vi "Overview Facade.vi"(0 "Data In":T4, 2 "Display State In":T2={"Numeric"=0.0, "Fill Plots"=FALSE, "Cursor Redraw"=TRUE, "XYGraph Refnum"=refnum}, 3 "Container State":T3) -> (6 "Data Out":T4, 7 "Display State Out":T2={"Numeric"=0.0, "Fill Plots"=FALSE, "Cursor Redraw"=TRUE, "XYGraph Refnum"=refnum}, 8 "Action":T1)   [LabVIEW 2020, in "Overview XControl.xctl"]
uses:
  Overview XControl.xctl
  Overview Data.ctl
  <vilib>/_xctls/Container State.ctl
  Overview State.ctl
  <vilib>/_xctls/Action.ctl
  <vilib>/Analysis/2dsp.llb/Decimate (single shot, DBL).vi
  <vilib>/_xctls/XControlSupport.lvlib
  <vilib>/Analysis/NI_AALPro.lvlib
panel:
  out "Overview":cluster{"X":dbl[], "Y":dbl[]}[](graph)
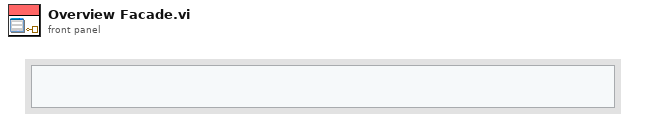
[diagram p1: front panel]
types:
  T1 = typedef "XControlSupport.lvlib/Action.ctl" = cluster{"Data Changed?":bool, "State Changed?":bool, "Action Name":string}
  T2 = typedef "Overview XControl.xctl/Overview State.ctl" = cluster{"Numeric":dbl, "Fill Plots":bool, "Cursor Redraw":bool, "XYGraph Refnum":refnum<vi>}
  T3 = typedef "XControlSupport.lvlib/Container State.ctl" = cluster{"Indicator?":bool, "Run Mode?":bool, " Refnum":refnum<vi>}
  T4 = typedef "Overview XControl.xctl/Overview Data.ctl" = cluster{"X":dbl[], "Y":dbl[]}[]
  T5 = enum16{"Move", "left cursor", "right cursor", "none"}
  T6 = cluster{"Decimated Array":dbl[], "Decimated Array":dbl[]}
  T7 = cluster{"Cursor Span":dbl, "Icon":u16, "Mouse Down":bool, "Owning VI":refnum<vi>, "Mouse area":enum16{"Move", "left cursor", "right cursor", "none"}, "Dragging":bool, "Drag Offset":dbl, "Original Cursor Pos":cluster{"Left":dbl, "Right":dbl, "Span":dbl}, "Cursor Redraw":bool}
  T8 = typedef "LVPoint32TypeDef.ctl" = cluster{"Horizontal":i32, "Vertical":i32}
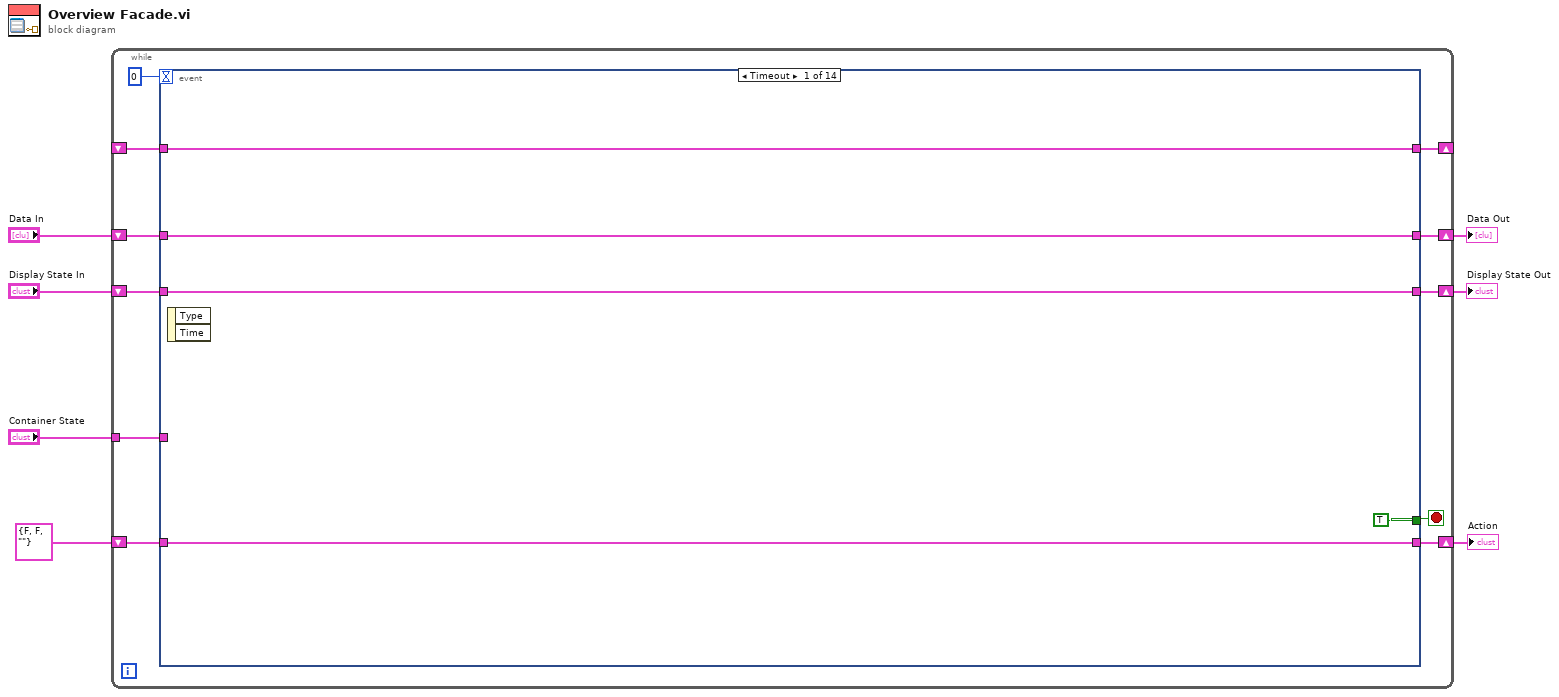
[diagram p0: block diagram]
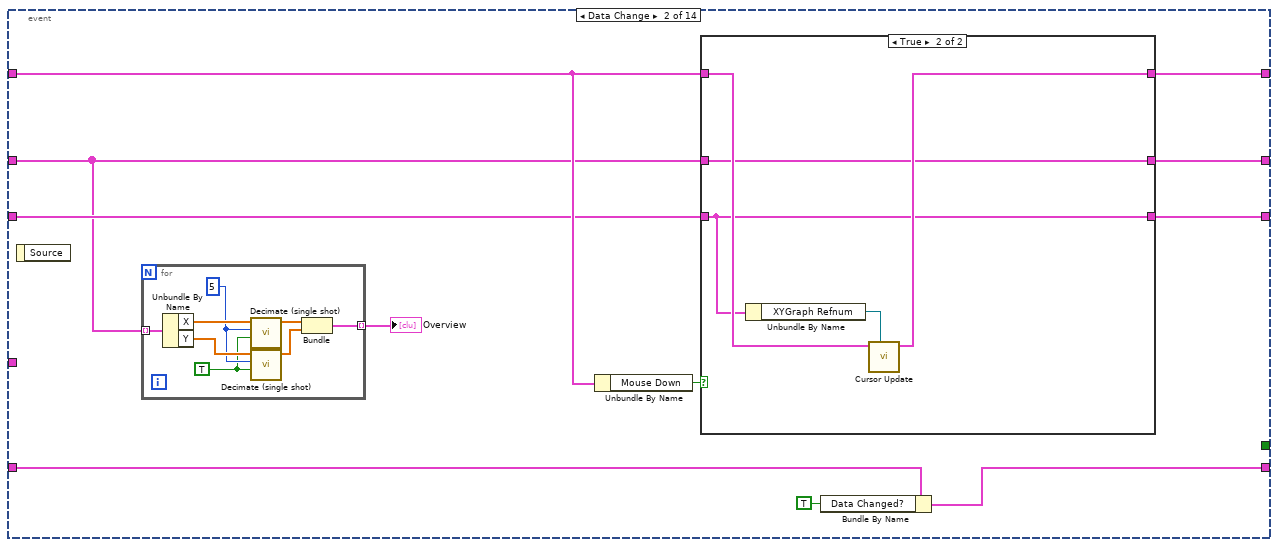
[diagram p2: hidden frame]
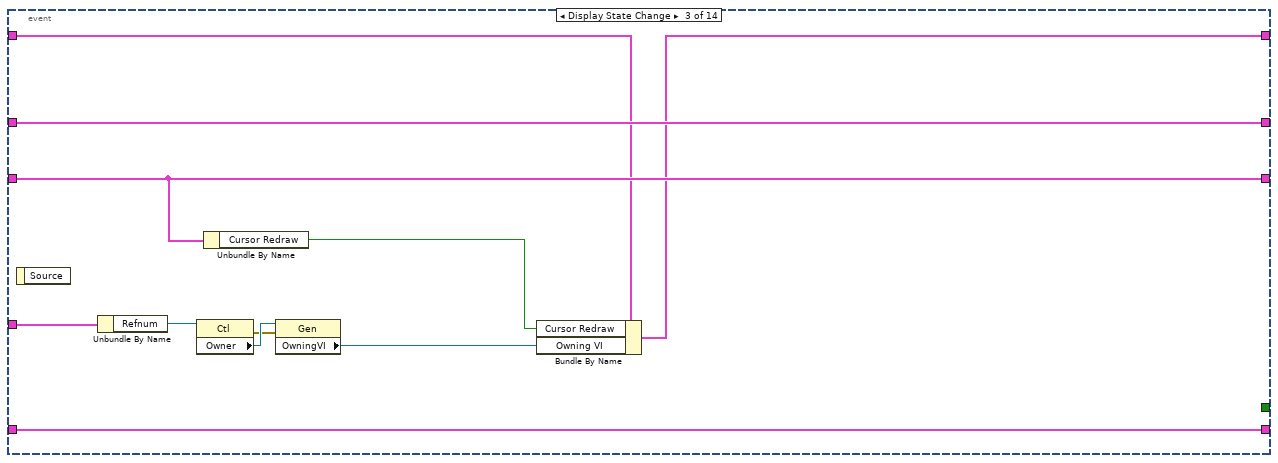
[diagram p4: hidden frame]
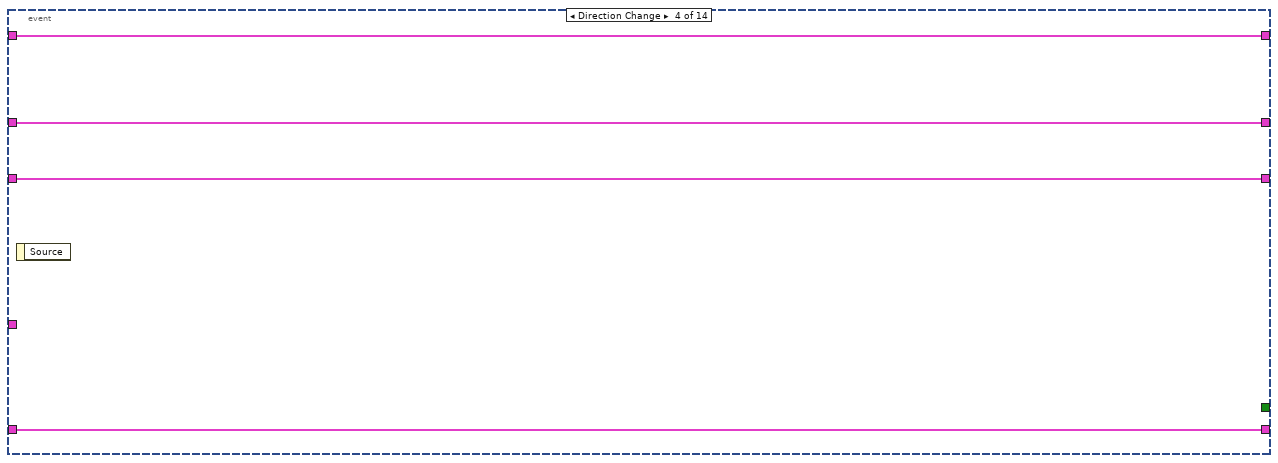
[diagram p5: hidden frame]
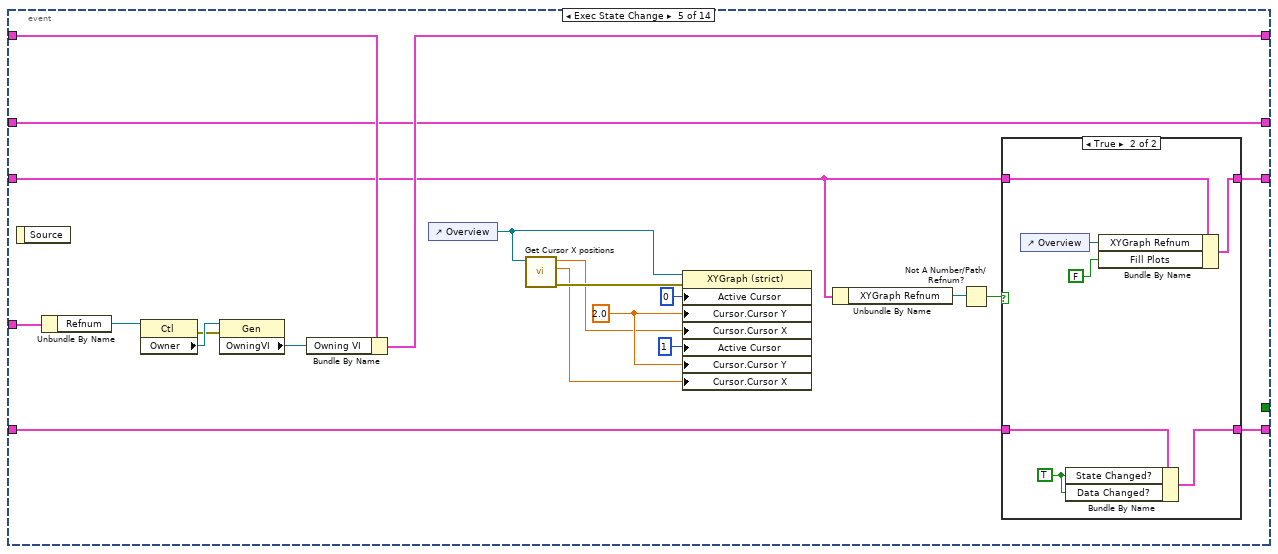
[diagram p6: hidden frame]
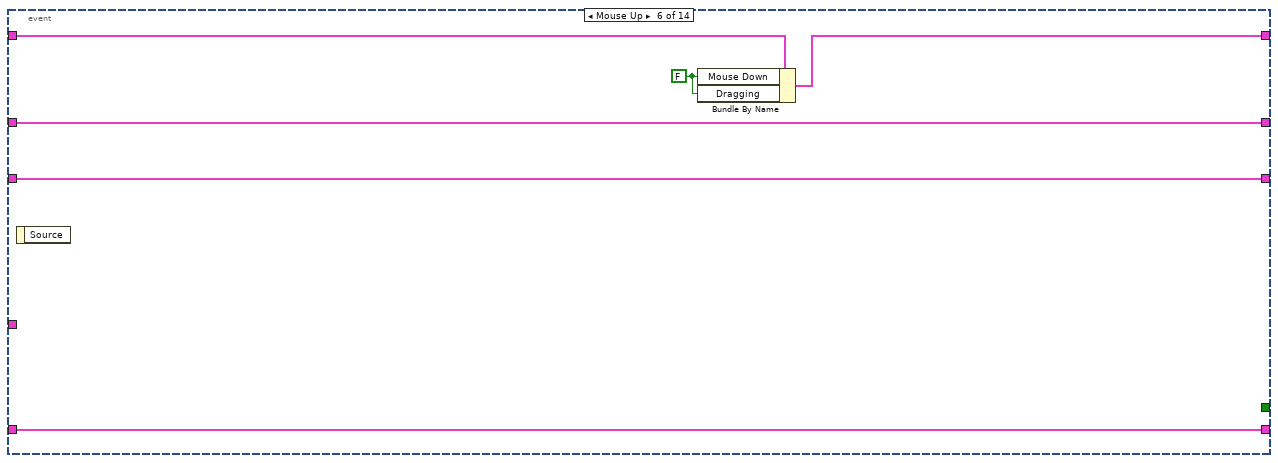
[diagram p8: hidden frame]
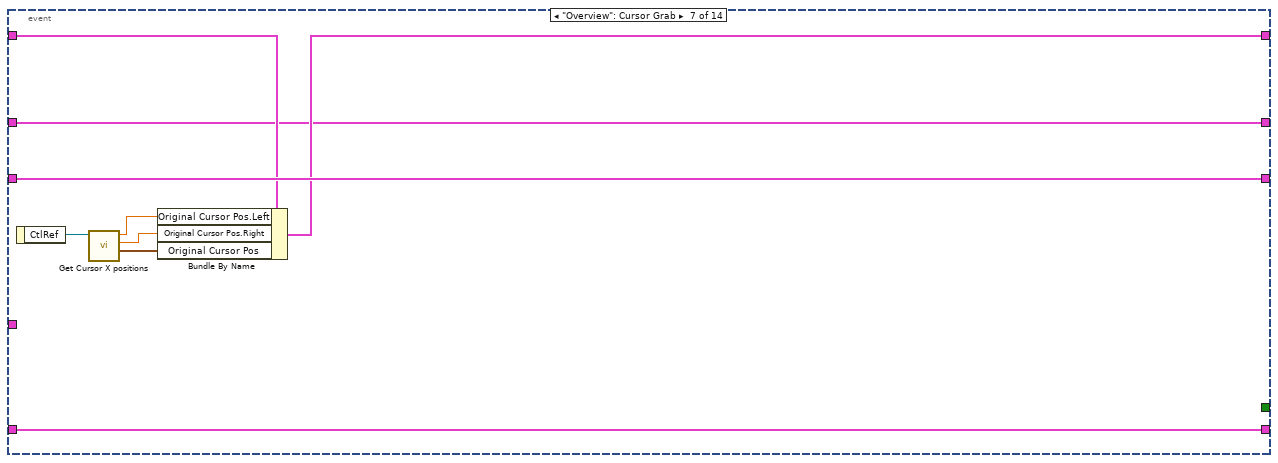
[diagram p9: hidden frame]
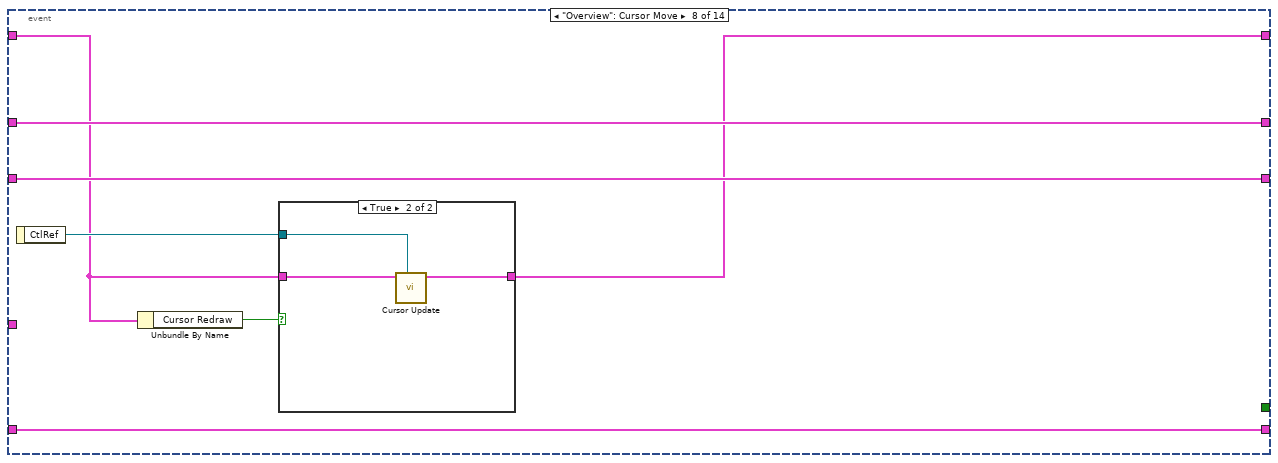
[diagram p10: hidden frame]
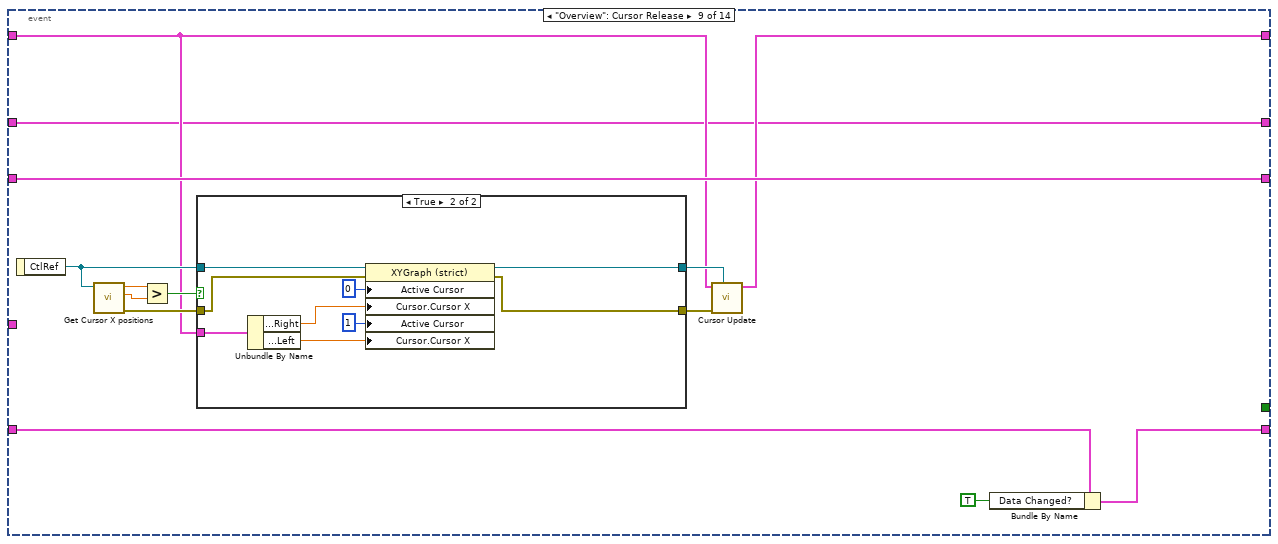
[diagram p12: hidden frame]
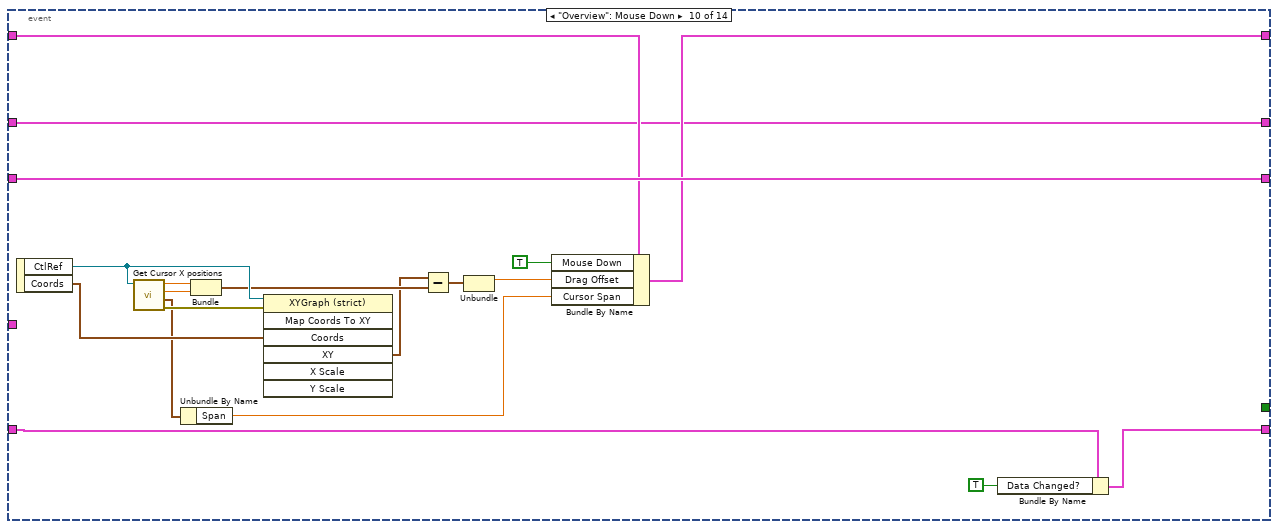
[diagram p14: hidden frame]
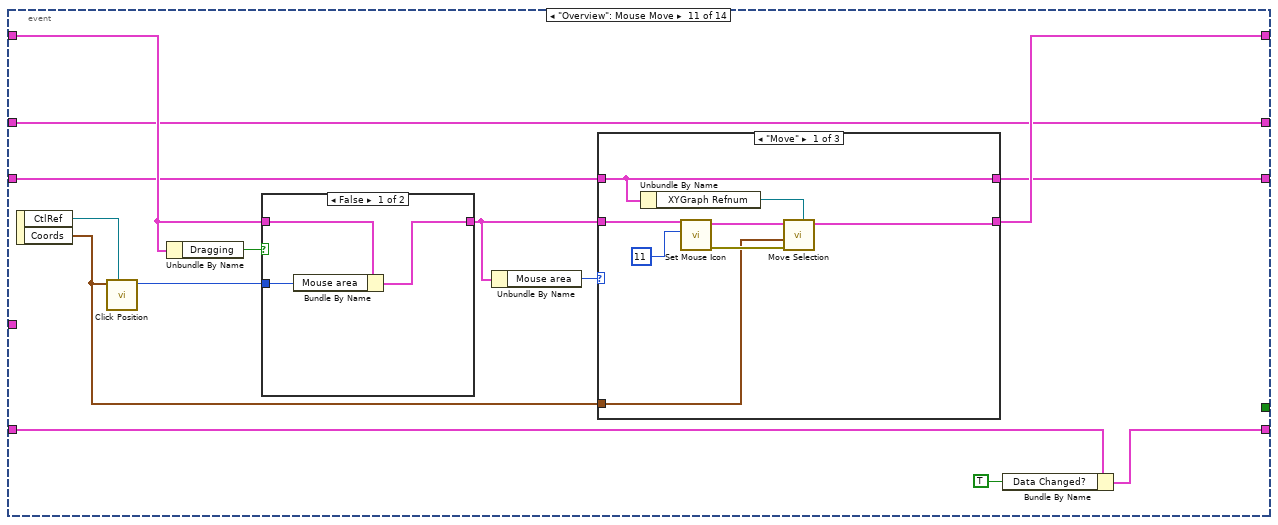
[diagram p15: hidden frame]
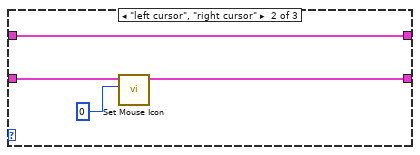
[diagram p16: hidden frame]
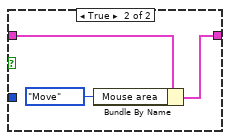
[diagram p18: hidden frame]
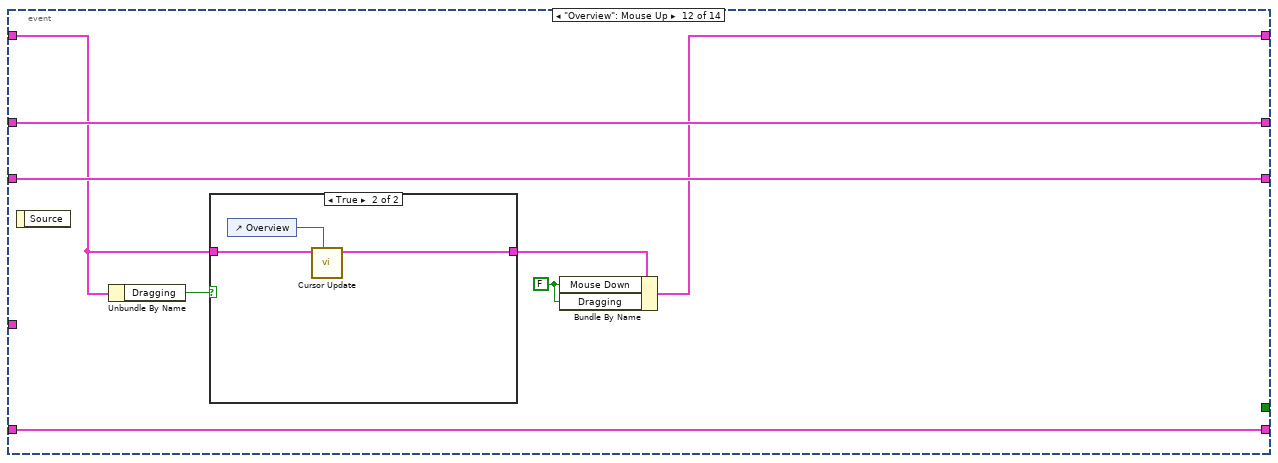
[diagram p19: hidden frame]
diagram:
  n1 = while {
    shift-right: [w17] -> w4
    shift-left: "Display State In" -> [w18]
    tunnel: "Container State" -> [w14]
    shift-right: [w12] -> w7
    shift-left: "Data In" -> [w13]
    shift-right: [w10] -> w2
    shift-left: T1 {"Data Changed?"=FALSE, "State Changed?"=FALSE, "Action Name"=""} ("Action") -> [w11]
    shift-right: [w9] -> _
    shift-left: _ -> [w8]
    stop <- w16 stop-if-true
    n2 = event shown="[0] Timeout" {
      selector: _ -> [_ _ _ _ _ _ _ _ _ _ _ _ _ _]
      dyn-events: _ -> [_ _ _ _ _ _ _ _ _ _ _ _ _ _]
      timeout: 0 -> [_ _ _ _ _ _ _ _ _ _ _ _ _ _]
      tunnel: w18 -> [w21 w27 w54 w63 w73 w101 w110 w117 w135 w165 w168 w207 w217 w226]
      tunnel: [w21 w26 w54 w63 w72 w101 w110 w117 w135 w165 w167 w207 w217 w226] -> w17
      tunnel: [TRUE _ _ _ _ _ _ _ _ _ _ _ _ _] -> w16
      tunnel: w14 -> [_ _ w55 _ w83 _ _ _ _ _ _ _ _ _]
      tunnel: w13 -> [w20 w25 w61 w65 w66 w100 w102 w116 w122 w147 w166 w206 w216 w218]
      tunnel: [w20 w28 w61 w65 w66 w100 w102 w116 w122 w147 w166 w206 w216 w218] -> w12
      tunnel: [w22 w32 w60 w64 w71 w99 w109 w115 w123 w148 w169 w205 w215 w225] -> w10
      tunnel: w11 -> [w22 w34 w60 w64 w74 w99 w109 w115 w124 w149 w170 w205 w215 w225]
      tunnel: [w19 w29 w52 w62 w80 w96 w105 w111 w126 w151 w172 w200 w212 w219] -> w9
      tunnel: w8 -> [w19 w31 w53 w62 w82 w97 w107 w112 w128 w152 w178 w203 w214 w219]
      event Timeout {
        n3 = event-data() -> ()  [unwired: 1 in, 2 out]
      }
      event Data Change {
        n4 = event-data() -> ()  [unwired: 1 in, 1 out]
        n5 = for {
          tunnel: w25 -> [w42] mode=indexing
          tunnel: [w35] -> w24 mode=indexing
          w38 = TRUE ("averaging")
          w39 = 5 ("decimating factor")
          n6 = Unbundle By Name(w42) -> ("X"=w41:dbl[], "Y"=w40:dbl[])
          n7 = call-poly <vilib>:"Decimate (single shot).vi"("averaging"=w38, "decimating factor"=w39, "X"=w41) -> ("Decimated Array"=w37:dbl[])  [unwired: 7 in, 1 out]
          n8 = call-poly <vilib>:"Decimate (single shot).vi"("averaging"=w38, "decimating factor"=w39, "X"=w40) -> ("Decimated Array"=w36:dbl[])  [unwired: 7 in, 1 out]
          n9 = Bundle("Decimated Array"=w37, "Decimated Array"=w36) -> (w35:T6)  [unwired: 1 in]
        }
        "Overview" <- w24
        n10 = Unbundle By Name(w31) -> ("Mouse Down"=w30:bool)
        n11 = case shown="True" w30 {
          tunnel: w31 -> [w45 w50]
          tunnel: [w45 w49] -> w29
          tunnel: w25 -> [w44 w46]
          tunnel: [w44 w46] -> w28
          tunnel: w27 -> [w43 w47]
          tunnel: [w43 w47] -> w26
          frame False {
          }
          frame True {
            n12 = Unbundle By Name(w47) -> ("XYGraph Refnum"=w48:refnum<vi>)
            n13 = call "Cursor Update.vi"("XY Graph Ref"=w48, "Xinformation In"=w50) -> ("Xinformation Out"=w49:T7)  [unwired: 8 in, 1 out]
          }
        }
        n14 = Bundle By Name(cluster=w34, "Data Changed?"=TRUE) -> (w32:T1)
      }
      event Display State Change {
        n15 = event-data() -> ()  [unwired: 1 in, 1 out]
        n16 = Unbundle By Name(w55) -> ("Refnum"=w58:refnum<vi>)
        n17 = property class="Ctl"(reference=w58) -> (error out=w57:errorcluster, "Owner"=w59:refnum<vi>)  [unwired: 1 in, 1 out]
        n18 = Unbundle By Name(w54) -> ("Cursor Redraw"=w51:bool)
        n19 = property class="Gen"(reference=w59, error in=w57) -> ("OwningVI"=w56:refnum<vi>)  [unwired: 2 out]
        n20 = Bundle By Name(cluster=w53, "Cursor Redraw"=w51, "Owning VI"=w56) -> (w52:T7)
      }
      event Direction Change {
        n21 = event-data() -> ()  [unwired: 1 in, 1 out]
      }
      event Exec State Change {
        w70 = 2.0
        n22 = event-data() -> ()  [unwired: 1 in, 1 out]
        n23 = Unbundle By Name(w83) -> ("Refnum"=w85:refnum<vi>)
        n24 = property class="Ctl"(reference=w85) -> (error out=w84:errorcluster, "Owner"=w86:refnum<vi>)  [unwired: 1 in, 1 out]
        n25 = property class="Gen"(reference=w86, error in=w84) -> ("OwningVI"=w81:refnum<vi>)  [unwired: 2 out]
        n26 = Bundle By Name(cluster=w82, "Owning VI"=w81) -> (w80:T7)
        n27 = control-ref of="Overview"() -> (w78:refnum<vi>)
        n28 = call "Get Cursor X positions.vi"("XY Graph Ref"=w78) -> ("error out"=w79:errorcluster, "Right"=w67:dbl, "Left"=w68:dbl)  [unwired: 7 in, 1 out]
        n29 = property class="XYGraph (strict)"(reference=w78, error in=w79, "Active Cursor"=u32 0, "Cursor.Cursor Y"=w70, "Cursor.Cursor X"=w68, "Active Cursor"=u32 1, "Cursor.Cursor Y"=w70, "Cursor.Cursor X"=w67) -> ()  [unwired: 2 out]
        n30 = Unbundle By Name(w73) -> ("XYGraph Refnum"=w76:refnum<vi>)
        n31 = Not A Number/Path/Refnum?(number/path/refnum=w76) -> (NaN/Path/Refnum?=w75:bool)
        n32 = case shown="True" w75 {
          tunnel: w74 -> [w87 w91]
          tunnel: w73 -> [w88 w95]
          tunnel: [w88 w92] -> w72
          tunnel: [w87 w90] -> w71
          frame False {
          }
          frame True {
            w89 = TRUE ("State Changed?")
            n33 = control-ref of="Overview"() -> (w94:refnum<vi>)
            n34 = Bundle By Name(cluster=w91, "State Changed?"=w89, "Data Changed?"=w89) -> (w90:T1)
            n35 = Bundle By Name(cluster=w95, "XYGraph Refnum"=w94, "Fill Plots"=FALSE) -> (w92:T2)
          }
        }
      }
      event Mouse Up {
        w98 = FALSE ("Mouse Down")
        n36 = event-data() -> ()  [unwired: 1 in, 1 out]
        n37 = Bundle By Name(cluster=w97, "Mouse Down"=w98, "Dragging"=w98) -> (w96:T7)
      }
      event "Overview": Cursor Grab {
        n38 = event-data() -> ("CtlRef"=w108:refnum<vi>)  [unwired: 1 in]
        n39 = call "Get Cursor X positions.vi"("XY Graph Ref"=w108) -> ("Cursors"=w106:cluster{"Left":dbl, "Right":dbl, "Span":dbl}, "Right"=w103:dbl, "Left"=w104:dbl)  [unwired: 7 in, 1 out]
        n40 = Bundle By Name(cluster=w107, "Original Cursor Pos.Left"=w104, "Original Cursor Pos.Right"=w103, "Original Cursor Pos"=w106) -> (w105:T7)
      }
      event "Overview": Cursor Move {
        n41 = event-data() -> ("CtlRef"=w113:refnum<vi>)  [unwired: 1 in]
        n42 = Unbundle By Name(w112) -> ("Cursor Redraw"=w114:bool)
        n43 = case shown="True" w114 {
          tunnel: w113 -> [_ w121]
          tunnel: w112 -> [w118 w120]
          tunnel: [w118 w119] -> w111
          frame False {
          }
          frame True {
            n44 = call "Cursor Update.vi"("XY Graph Ref"=w121, "Xinformation In"=w120) -> ("Xinformation Out"=w119:T7)  [unwired: 8 in, 1 out]
          }
        }
      }
      event "Overview": Cursor Release {
        n45 = event-data() -> ("CtlRef"=w134:refnum<vi>)  [unwired: 1 in]
        n46 = call "Get Cursor X positions.vi"("XY Graph Ref"=w134) -> ("error out"=w130:errorcluster, "Right"=w132:dbl, "Left"=w133:dbl)  [unwired: 7 in, 1 out]
        n47 = Greater?(x=w133, y=w132) -> (0:w131:bool)
        n48 = case shown="True" w131 {
          tunnel: w134 -> [w137 w142]
          tunnel: w130 -> [w136 w141]
          tunnel: [w137 w140] -> w129
          tunnel: w128 -> [_ w139]
          tunnel: [w136 w138] -> w127
          frame False {
          }
          frame True {
            n49 = Unbundle By Name(w139) -> ("Original Cursor Pos.Right"=w145:dbl, "Original Cursor Pos.Left"=w146:dbl)
            n50 = property class="XYGraph (strict)"(reference=w142, error in=w141, "Active Cursor"=u32 0, "Cursor.Cursor X"=w145, "Active Cursor"=u32 1, "Cursor.Cursor X"=w146) -> (reference out=w140:refnum<vi>, error out=w138:errorcluster)
          }
        }
        n51 = call "Cursor Update.vi"("XY Graph Ref"=w129, "error in (no error)"=w127, "Xinformation In"=w128) -> ("Xinformation Out"=w126:T7)  [unwired: 7 in, 1 out]
        n52 = Bundle By Name(cluster=w124, "Data Changed?"=TRUE ("State Changed?")) -> (w123:T1)
      }
      event "Overview": Mouse Down {
        n53 = event-data() -> ("CtlRef"=w163:refnum<vi>, "Coords"=w162:T8)  [unwired: 1 in]
        n54 = call "Get Cursor X positions.vi"("XY Graph Ref"=w163) -> ("error out"=w164:errorcluster, "Cursors"=w154:cluster{"Left":dbl, "Right":dbl, "Span":dbl}, "Right"=w160:dbl, "Left"=w161:dbl)  [unwired: 7 in]
        n55 = Unbundle By Name(w154) -> ("Span"=w153:dbl)
        n56 = Bundle("Left"=w161, "Right"=w160) -> (w159:cluster{"Left":dbl, "Right":dbl})  [unwired: 1 in]
        n57 = invoke on="Invoke Node" class="XYGraph (strict)" method="Map Coords To XY"(reference=w163, error in=w164, "Coords"=w162) -> ("XY"=w158:cluster{"X":dbl, "Y":dbl})  [unwired: 4 in, 6 out]
        n58 = Subtract(x=w158, y=w159) -> (x-y=w155:cluster{dbl, dbl})
        n59 = Unbundle(w155) -> (w157:dbl)  [unwired: 1 out]
        n60 = Bundle By Name(cluster=w152, "Mouse Down"=TRUE, "Drag Offset"=w157, "Cursor Span"=w153) -> (w151:T7)
        n61 = Bundle By Name(cluster=w149, "Data Changed?"=TRUE ("State Changed?")) -> (w148:T1)
      }
      event "Overview": Mouse Move {
        n62 = event-data() -> ("CtlRef"=w173:refnum<vi>, "Coords"=w175:T8)  [unwired: 1 in]
        n63 = call "Click Position.vi"("XY Graph Ref"=w173, "Click Coords"=w175) -> ("Operation"=w174:T5)  [unwired: 8 in, 1 out]
        n64 = Unbundle By Name(w178) -> ("Dragging"=w179:bool)
        n65 = case shown="False" w179 {
          tunnel: w178 -> [w196 w199]
          tunnel: w174 -> [w195 _]
          tunnel: [w194 w197] -> w176
          frame False {
            n66 = Bundle By Name(cluster=w196, "Mouse area"=w195) -> (w194:T7)
          }
          frame True {
            n67 = Bundle By Name(cluster=w199, "Mouse area"=T5."Move") -> (w197:T7)
          }
        }
        n68 = Unbundle By Name(w176) -> ("Mouse area"=w177:T5)
        n69 = case shown="\"Move\"" w177 {
          tunnel: w176 -> [w186 w191 w193]
          tunnel: [w183 w189 w193] -> w172
          tunnel: w175 -> [w182 _ _]
          tunnel: w168 -> [w181 w188 w192]
          tunnel: [w181 w188 w192] -> w167
          frame "Move" {
            n70 = Unbundle By Name(w181) -> ("XYGraph Refnum"=w180:refnum<vi>)
            n71 = call "Set Mouse Icon.vi"("icon"=u16 11, "Xinformation In"=w186) -> ("error out"=w185:errorcluster, "Xinformation Out"=w184:T7)  [unwired: 8 in]
            n72 = call "Move Selection.vi"("XY Graph Ref"=w180, "error in (no error)"=w185, "Coords"=w182, "Xinformation In"=w184) -> ("Xinformation Out"=w183:T7)  [unwired: 6 in, 1 out]
          }
          frame "left cursor", "right cursor" {
            n73 = call "Set Mouse Icon.vi"("icon"=u16 0, "Xinformation In"=w191) -> ("Xinformation Out"=w189:T7)  [unwired: 8 in, 1 out]
          }
          frame "none", Default {
          }
        }
        n74 = Bundle By Name(cluster=w170, "Data Changed?"=TRUE ("State Changed?")) -> (w169:T1)
      }
      event "Overview": Mouse Up {
        w202 = FALSE
        n75 = event-data() -> ()  [unwired: 1 in, 1 out]
        n76 = Unbundle By Name(w203) -> ("Dragging"=w204:bool)
        n77 = case shown="True" w204 {
          tunnel: w203 -> [w208 w211]
          tunnel: [w208 w209] -> w201
          frame False {
          }
          frame True {
            n78 = control-ref of="Overview"() -> (w210:refnum<vi>)
            n79 = call "Cursor Update.vi"("XY Graph Ref"=w210, "Xinformation In"=w211) -> ("Xinformation Out"=w209:T7)  [unwired: 8 in, 1 out]
          }
        }
        n80 = Bundle By Name(cluster=w201, "Mouse Down"=w202, "Dragging"=w202) -> (w200:T7)
      }
      event "Overview": Mouse Leave {
        n81 = event-data() -> ()  [unwired: 1 in, 1 out]
        n82 = call "Set Mouse Icon.vi"("icon"=u16 0, "Xinformation In"=w214) -> ("Xinformation Out"=w212:T7)  [unwired: 8 in, 1 out]
      }
      event "Overview": Scale Range Change {
        n83 = event-data() -> ("CtlRef"=w224:refnum<vi>)  [unwired: 1 in]
        n84 = Unbundle By Name(w219) -> ("Original Cursor Pos.Left"=w221:dbl, "Original Cursor Pos.Right"=w220:dbl)
        n85 = property class="XYGraph (strict)"(reference=w224, "Active Cursor"=u32 0, "Cursor.Cursor X"=w221, "Active Cursor"=u32 1, "Cursor.Cursor X"=w220) -> ()  [unwired: 1 in, 2 out]
      }
    }
  }
  "Display State Out" <- w4
  "Data Out" <- w7
  "Action" <- w2
